vi "Vanna Global.vi"() -> ()   [LabVIEW 2019]
uses:
  Vanna Mode Type Def.ctl
  Vanna Command Type Def.ctl
panel:
  in  "Vanna Command Done?":cluster{"Done?":bool, "Timestamp (ms)":dbl}
  in  "Vanna Command":T1
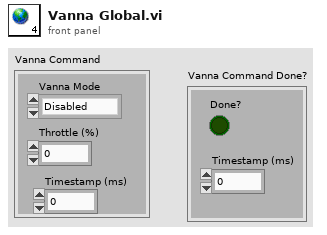
[diagram p1: front panel]
types:
  T1 = typedef "Vanna Command Type Def.ctl" = cluster{"Vanna Mode":T2, "Throttle (%)":dbl, "Timestamp (ms)":dbl}
  T2 = typedef "Vanna Mode Type Def.ctl" = enum16{"Disabled", "Raw Throttle", "Rotation Control", "Position Control"}
diagram:
